vi "NewMaze.vi"(8 "error in (no error)":errorcluster) -> (0 "error out":errorcluster, 3 "Maze":refnum<class "Maze.lvclass">)   [LabVIEW 2020, in "Maze.lvclass"]
uses:
  Maze.lvclass
  Maze.lvclass/Maze.ctl
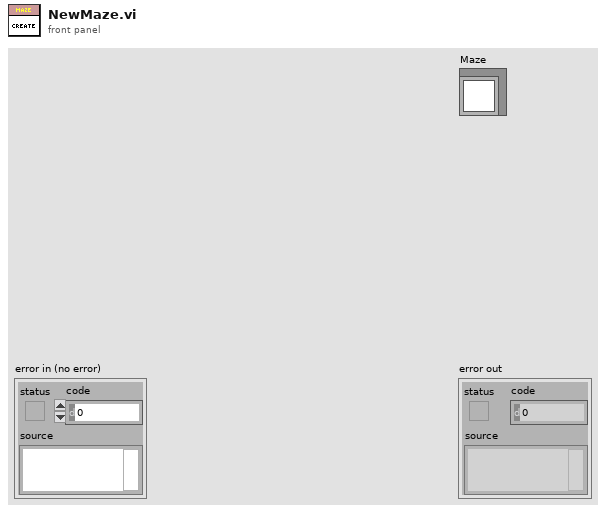
[diagram p1: front panel]
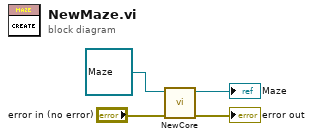
[diagram p0: block diagram]
diagram:
  n1 = call-dynamic "NewCore.vi"("error in (no error)"="error in (no error)", "Maze"=refnum<class "Maze.lvclass"> refnum) -> ("error out"=→"error out":errorcluster, "Maze"=→"Maze":refnum<class "Maze.lvclass">)  [unwired: 8 in]
